vi "Get Reference.vi"(8 "error in (no error)":errorcluster, 11 "Credit Transaction in":refnum<class "Credit Transaction.lvclass">) -> (0 "error out":errorcluster, 2 "Ref":string, 3 "Credit Transaction out":refnum<class "Credit Transaction.lvclass">)   [LabVIEW 2018, in "Credit Transaction.lvclass"]
uses:
  Credit Transaction.lvclass
  Credit Transaction.lvclass/Credit Transaction.ctl
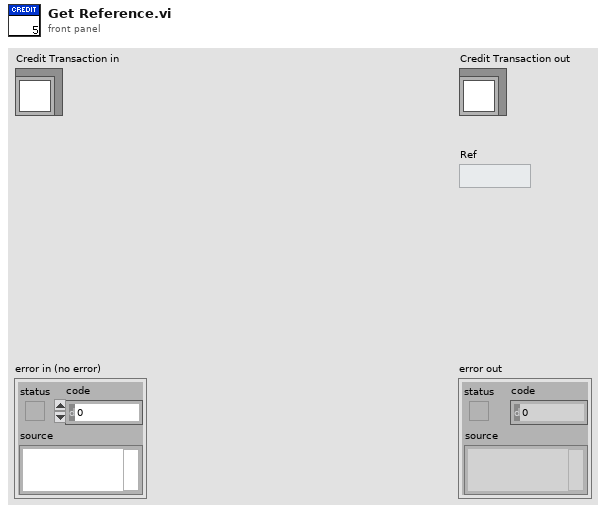
[diagram p1: front panel]
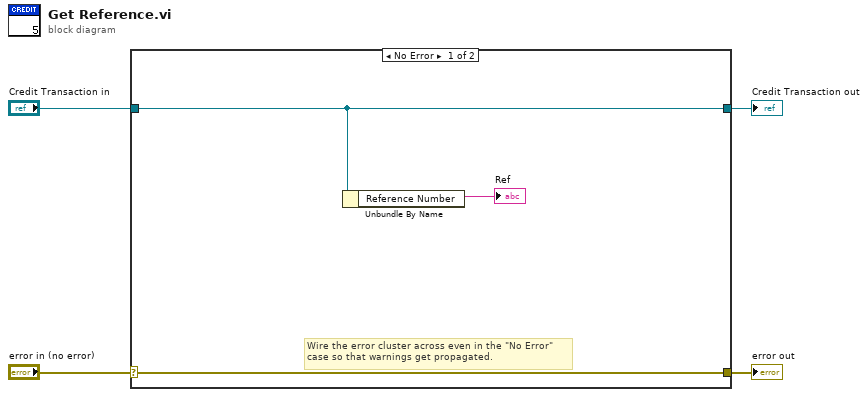
[diagram p0: block diagram]
diagram:
  n1 = case shown="No Error" "error in (no error)" {
    selector: "error in (no error)" -> [w7 w9]
    tunnel: [w7 w9] -> w3
    tunnel: [w6 w8] -> w1
    tunnel: "Credit Transaction in" -> [w6 w8]
    frame No Error {
      # "Wire the error cluster across even in the \"No Error\"\ncase so that warnings get propagated."
      n2 = Unbundle By Name(w6) -> ("Reference Number"=→"Ref":string)
    }
    frame Error {
    }
  }
  "error out" <- w3
  "Credit Transaction out" <- w1
